vi "电机ID计算.vi"(1 "电机ID":string="01", 2 "主机id":string="00fd", 3 "通信模式":string="01") -> (0 "最终输出报文":string)   [LabVIEW 2023]
panel:
  out "连接为字符串":string
  out "16进制转换10进制":u32
  out "十进制数":i32
  out "检验转为16进制":string
  out "左移3位加100":string
  out "二进制转换":string
  # "00fd是主机地址"
  # "运控模式 01"
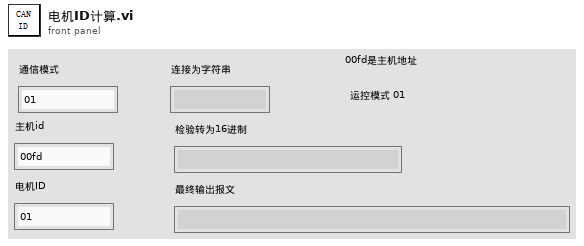
[diagram p1: front panel]
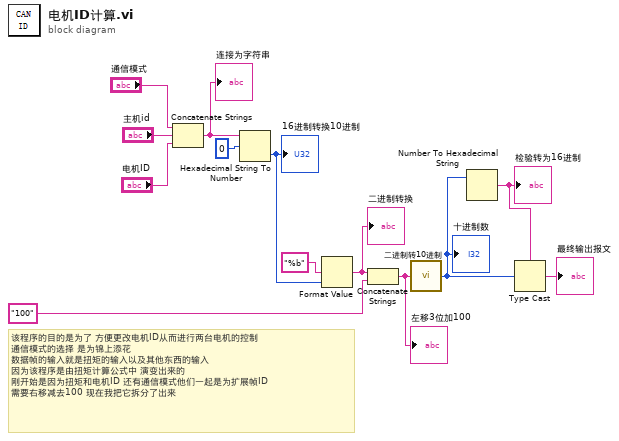
[diagram p0: block diagram]
diagram:
  # "该程序的目的是为了 方便更改电机ID从而进行两台电机的控制 \n通信模式的选择 是为锦上添花 \n数据帧的输入就是扭矩的输入以及其他东西的输入\n因为该程序是由扭矩计算公式中 演变出来的\n刚开始是因为扭矩和电机ID 还有通信模式他们一起是为扩展帧ID\n需要右移减去100 现在我把它拆分了出来"
  n1 = Concatenate Strings("通信模式", "主机id", "电机ID") -> (w2:string)
  "连接为字符串" <- w2
  n2 = Hexadecimal String To Number(string=w2, offset=0 ("偏移量")) -> (number=w6:u32)  [unwired: 1 in, 1 out]
  "16进制转换10进制" <- w6
  n3 = Format Value(format string="%b" ("格式字符串"), value (0)=w6) -> (output string=w9:string)  [unwired: 1 in]
  "二进制转换" <- w9
  n4 = Concatenate Strings(w9, "100" ("字符串")) -> (w8:string)
  "左移3位加100" <- w8
  n5 = call "二进制转10进制.vi"("字符串"=w8) -> ("十进制数"=w12:i32)
  "十进制数" <- w12
  n6 = Number To Hexadecimal String(2:w12) -> (0:w11:string)  [unwired: 1 in]
  "检验转为16进制" <- w11
  n7 = Type Cast(type=w11, x=w12) -> (*(type *) &x=→"最终输出报文":string)
